vi "_Set Splitter Properties.vi"(8 "error in (no error)":errorcluster, 10 "Splitter Properties":T1, 11 "Item_Refnums_Array":T2[](array[typedef])) -> (0 "error out":errorcluster, 3 "Item_Refnums_Array Out":T2[](array[typedef]))   [LabVIEW 2013, in "UI Panels.lvlib" / "Panels_XControl.xctl"]
uses:
  Panels_XControl.xctl
  Controls/References/Panel_Refnums.ctl
  Controls/Panel_Command_Enum.ctl
  Typedefs/Splitter Properties.ctl
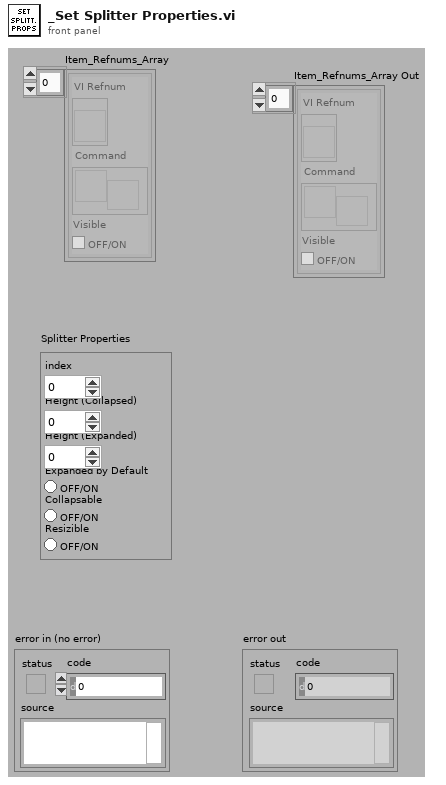
[diagram p1: front panel]
types:
  T1 = typedef "UI Panels.lvlib/Panels_XControl.xctl/Splitter Properties.ctl" = cluster{"index":i32, "Height (Collapsed)":i32, "Height (Expanded)":i32, "Expanded by Default":bool, "Collapsable":bool, "Resizible":bool}
  T2 = typedef "UI Panels.lvlib/Panels_XControl.xctl/Panel_Refnums.ctl" = cluster{"VI Refnum":refnum<vi>, "Command":refnum<user-event>, "Visible":bool}
  T3 = typedef "UI Panels.lvlib/Panels_XControl.xctl/Panel_Command_Enum.ctl" = enum16{"Idle", "Remove & Stop", "Add Item", "Delete Item", "Delete All", "Insert into Subpanel", "Register Menu Events", "Update Value", "Remove from Subpanel", "Set Title", "Set Menu Items", "Insert SubPanel", "Set Splitter Position", "Set Splitter Properties", "Add Menu Items"}
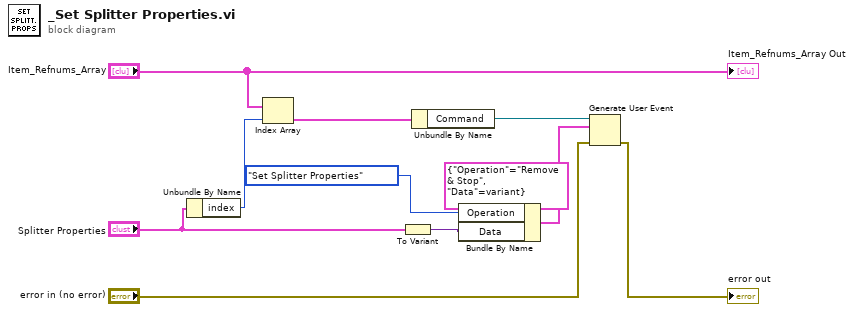
[diagram p0: block diagram]
diagram:
  n1 = Unbundle By Name("Splitter Properties") -> ("index"=w5:i32)
  n2 = Index Array(array="Item_Refnums_Array", index=w5) -> (element=w8:T2)
  n3 = To Variant(anything="Splitter Properties") -> (Variant=w7:variant)
  n4 = Unbundle By Name(w8) -> ("Command"=w4:refnum<user-event>)
  n5 = Bundle By Name(cluster=cluster{"Operation":T3, "Data":variant} {"Operation"=enum."Remove & Stop", "Data"=variant} ("Item_Command"), "Operation"=Panel_Command_Enum."Set Splitter Properties", "Data"=w7) -> (w3:cluster{"Operation":T3, "Data":variant})
  n6 = Generate User Event(user event=w4, event data cluster=w3, error in="error in (no error)") -> (error out=→"error out":errorcluster)  [unwired: 1 in, 1 out]
  "Item_Refnums_Array Out" <- "Item_Refnums_Array"
